vi "Memory.Pointer.Numeric.Read.Safe (U64).vi"(8 "error in (no error)":errorcluster, 10 "value":u64, 11 "Numeric Pointer in":refnum<class "Memory.Pointer.Numeric.lvclass">) -> (0 "error out":errorcluster, 2 "value out":u64, 3 "Numeric Pointer out":refnum<class "Memory.Pointer.Numeric.lvclass">)   [LabVIEW 2016, in "LabVIEW Memory Manager.lvlib" / "Memory.Pointer.Numeric.lvclass"]
uses:
  Memory.Pointer.Numeric.lvclass
  C:/Users/Ryan/Documents/Git/Sourcetree/LabVIEW-Memory-Manager/Source/Library/Classes/Pointer/Pointer.Void/Memory.Pointer.Void.lvclass
  Pointer.Void/Memory.Pointer.Void.lvclass/Memory.Pointer.Void.ctl
  Pointer.Void/Memory.Pointer.Void.lvclass
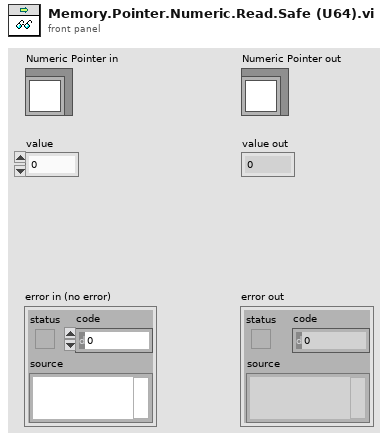
[diagram p1: front panel]
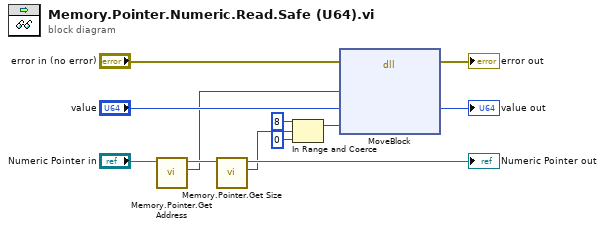
[diagram p0: block diagram]
diagram:
  n1 = call "Memory.Pointer.Get Address.vi"("Pointer in"="Numeric Pointer in") -> ("address"=w6:u64, "Pointer out"=w7:refnum<class "Memory.Pointer.Numeric.lvclass">)  [unwired: 8 in, 1 out]
  n2 = call "Memory.Pointer.Get Size.vi"("Pointer in"=w7) -> ("size"=w4:u64, "Pointer out"=→"Numeric Pointer out":refnum<class "Memory.Pointer.Numeric.lvclass">)  [unwired: 8 in, 1 out]
  n3 = In Range and Coerce(upper limit=u64 8, x=w4, lower limit=u64 0) -> (coerced(x)=w3:u64)  [unwired: 1 out]
  n4 = dll-call lib="LabVIEW" fn="MoveBlock"(error in="error in (no error)", "src"=w6, "dst"="value", "size"=w3) -> (error out=→"error out":errorcluster, "dst"=→"value out":u64)  [unwired: 5 in, 1 out]
